vi "Order_Items.vi"(7 "error in":errorcluster, 9 "State in":T1 caption="State", 10 "MCListbox Refnum in":refnum<vi>) -> (0 "error out":errorcluster, 2 "State out":T1 caption="State", 3 "MCListbox Refnum out":refnum<vi>)   [LabVIEW 2012, in "ListBox_XControl.xctl"]
doc: "Sort item names in the list box by column in either ascending or descending mode (alphabetically). \nSorted column header is bolded with a directional symbol \\/ or /\\"
uses:
  ListBox_XControl.xctl
  ListBox_State.ctl
  Order Type Def.ctl
  Value Filters.ctl
  <vilib>/Utility/miscctls.llb/LVRowAndColumnTypeDef.ctl
  <userlib>/_OpenG.lib/array/array.llb/Sort 2D Array (String)__ogtk.vi
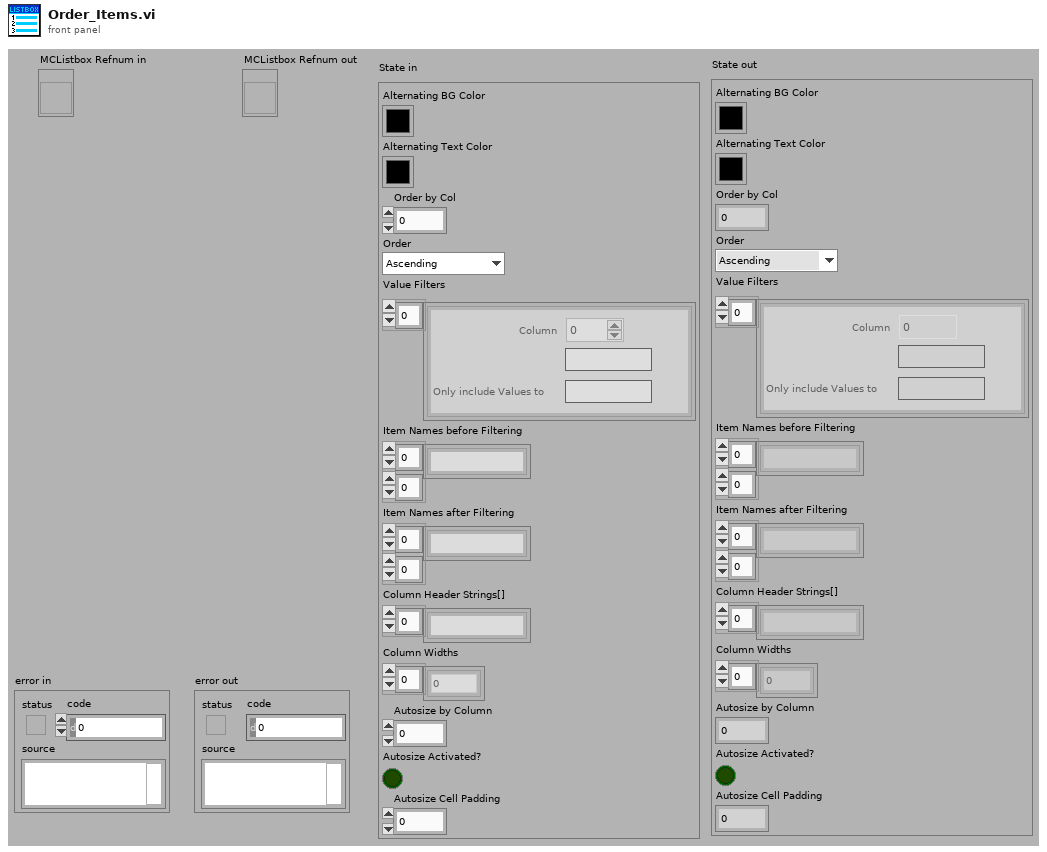
[diagram p1: front panel]
types:
  T1 = typedef "ListBox_XControl.xctl/ListBox_State.ctl" = cluster{"Alternating BG Color":u32, "Alternating Text Color":u32, "Order by Col":i32, "Order":T2, "Value Filters":T3, "Item Names before Filtering":string[][], "Item Names after Filtering":string[][], "Column Header Strings[]":string[], "Column Widths":u32[], "Autosize by Column":i32, "Autosize Activated?":bool, "Autosize Cell Padding":u32}
  T2 = typedef "ListBox_XControl.xctl/Order Type Def.ctl" = enum16{"Ascending", "Descending", "Off"}
  T3 = typedef "ListBox_XControl.xctl/Value Filters.ctl" = cluster{"Column":i32, "Only include Values From":string, "Only include Values to":string}[]
  T4 = typedef "LVRowAndColumnTypeDef.ctl" = cluster{"Row":i32, "Column":i32}
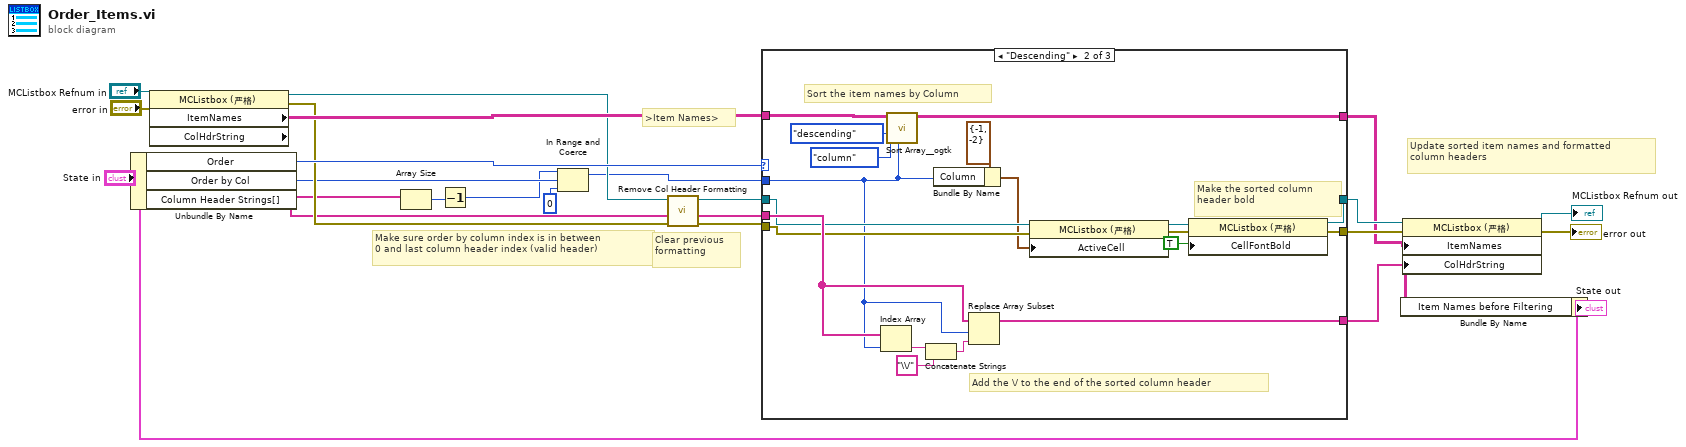
[diagram p0: block diagram]
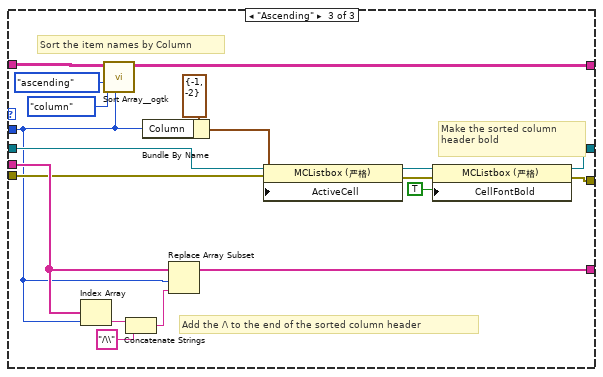
[diagram p3: hidden frame]
diagram:
  # "Clear previous\nformatting"
  # "Make sure order by column index is in between\n0 and last column header index (valid header)"
  # "Update sorted item names and formatted\ncolumn headers"
  # ">Item Names>"
  n1 = Unbundle By Name("State in") -> ("Order"=w22:T2, "Order by Col"=w9:i32, "Column Header Strings[]"=w4:string[])
  n2 = property on="Property Node" class="MCListbox (严格)" props=["ItemNames", "ColHdrString"](reference="MCListbox Refnum in", error in="error in") -> (reference out=w10:refnum<vi>, error out=w12:errorcluster, "ItemNames"=w21:string[][])  [unwired: 1 out]
  n3 = Array Size(array=w4) -> (size(s)=w7:i32)
  n4 = Decrement(x=w7) -> (x-1=w6:i32)
  n5 = In Range and Coerce(upper limit=w6, x=w9, lower limit=0) -> (coerced(x)=w5:i32)  [unwired: 1 out]
  n6 = call "Remove Col Header Formatting.vi"("error in"=w12, "Column Header Strings[] in"=w4, "MCListbox Refnum in"=w10) -> ("error out"=w11:errorcluster, "Column Header Strings[] out"=w15:string[])  [unwired: 6 in, 1 out]
  n7 = case shown="\"Descending\"" w22 {
    tunnel: w21 -> [w26 w44 w63]
    tunnel: w5 -> [_ w33 w46]
    tunnel: [w26 w42 w61] -> w1
    tunnel: w15 -> [w25 w38 w60]
    tunnel: [w25 w37 w56] -> w16
    tunnel: w10 -> [w24 w36 w50]
    tunnel: [w24 w31 w49] -> w14
    tunnel: w11 -> [w23 w35 w51]
    tunnel: [w23 w27 w48] -> w13
    frame "Off", Default {
      # "Sorting is turned off"
    }
    frame "Descending" {
      # "Make the sorted column\nheader bold"
      # "Sort the item names by Column"
      # "Add the \\/ to the end of the sorted column header"
      n8 = Index Array(array=w38, index=w33) -> (element=w41:string)
      n9 = call-poly <userlib>:"Sort Array__ogtk.vi"("Column/Row to Sort By"=w33, "Sort By in"=enum16{"row", "column"}."column", "Order"=enum16{"ascending", "descending"}."descending", "Array in"=w44) -> ("Sorted Array out"=w42:string[][])  [unwired: 4 in, 3 out]
      n10 = Concatenate Strings(w41, "\\/" ("string")) -> (w39:string)
      n11 = Bundle By Name(cluster=T4 {"Row"=-1, "Column"=-2} ("Active Cell:Active Cell"), "Column"=w33) -> (w32:T4)
      n12 = Replace Array Subset(array=w38, new element=w39, index=w33) -> (w37:string[])
      n13 = property on="Property Node" class="MCListbox (严格)"(reference=w36, error in=w35, "ActiveCell"=w32) -> (reference out=w30:refnum<vi>, error out=w29:errorcluster)
      n14 = property on="Property Node" class="MCListbox (严格)"(reference=w30, error in=w29, "CellFontBold"=TRUE ("Active Cell:Cell Font:Bold")) -> (reference out=w31:refnum<vi>, error out=w27:errorcluster)
    }
    frame "Ascending" {
      # "Make the sorted column\nheader bold"
      # "Sort the item names by Column"
      # "Add the /\\ to the end of the sorted column header"
      n15 = Index Array(array=w60, index=w46) -> (element=w59:string)
      n16 = call-poly <userlib>:"Sort Array__ogtk.vi"("Column/Row to Sort By"=w46, "Sort By in"=enum16{"row", "column"}."column", "Order"=enum16{"ascending", "descending"}."ascending", "Array in"=w63) -> ("Sorted Array out"=w61:string[][])  [unwired: 4 in, 3 out]
      n17 = Concatenate Strings(w59, "/\\" ("string")) -> (w57:string)
      n18 = Bundle By Name(cluster=T4 {"Row"=-1, "Column"=-2} ("Active Cell:Active Cell"), "Column"=w46) -> (w47:T4)
      n19 = Replace Array Subset(array=w60, new element=w57, index=w46) -> (w56:string[])
      n20 = property on="Property Node" class="MCListbox (严格)"(reference=w50, error in=w51, "ActiveCell"=w47) -> (reference out=w54:refnum<vi>, error out=w53:errorcluster)
      n21 = property on="Property Node" class="MCListbox (严格)"(reference=w54, error in=w53, "CellFontBold"=TRUE ("Active Cell:Cell Font:Bold")) -> (reference out=w49:refnum<vi>, error out=w48:errorcluster)
    }
  }
  n22 = Bundle By Name(cluster="State in", "Item Names before Filtering"=w1) -> (→"State out":T1)
  n23 = property on="Property Node" class="MCListbox (严格)"(reference=w14, error in=w13, "ItemNames"=w1, "ColHdrString"=w16) -> (reference out=→"MCListbox Refnum out":refnum<vi>, error out=→"error out":errorcluster)
